vi "Standalone Status Monitor.vi"(11 "configuration file path":path) -> ()   [LabVIEW 2017, in "Status Monitor Library.lvlib"]
doc: "Use this template to build a producer/consumer design pattern. Use this template when you need to execute a process, such as data analysis, when a data source, such as a triggered acquisition, produces data at an uneven rate and you need to execute the process when the data becomes available."
uses:
  Status Monitor Library.lvlib
  Communications/Communications Library.lvlib
  Network Shared Variables/Shared Variables Library.lvlib
panel:
  in  "Process Stop Button":bool
  out "Demuxing":bool
  out "Total Samples":i32
  out "Post-Buffered Samples":i32
  out "Pre-Buffered Samples":i32
  out "Device State":T1(ring)
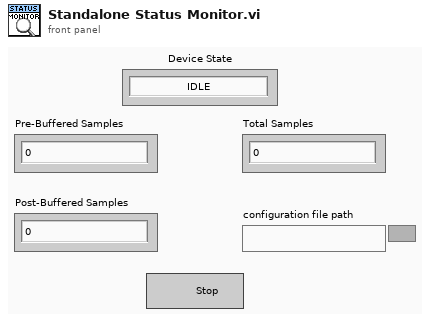
[diagram p1: front panel]
types:
  T1 = enum16{"IDLE", "ARM", "RUN_PRE-TRIGGER", "RUN_POST-TRIGGER", "POST_PROCESS", "CLEANUP"}
  T2 = typedef "Communications Library.lvlib/DTACQ Module Carrier Configuration--Cluster.ctl" = cluster{"Name":string, "IP":string, "Control Port":i32, "Timeout (ms)":i32, "Continuous Capture Port (Multiplexed)":i32, "Start HIL Shot Port":i32, "AWG Upload Port (Multiplexed)":i32, "Download Captured Data Port (Multiplexed)":i32, "Module Slots":i32, "Module Configurations":T3[]}
  T3 = typedef "Communications Library.lvlib/DTACQ Module Configuration--Cluster.ctl" = cluster{"Name":string, "Position":string, "Module Type":T4, "Control Port":i32, "Timeout (ms)":i32, "Channels":i32}
  T4 = typedef "Communications Library.lvlib/DTACQ Device Type--Enum.ctl" = enum16{"Carrier", "Analog In Module", "Analog Out Module", "Generic Module"}
  T5 = typedef "Communications Library.lvlib/DTACQ Connection Data--Cluster.ctl" = cluster{"Description":string, "Address":string, "Port":u16, "timeout (ms)":i32, "Termination Character":string, "TCP Connection Reference":refnum<k5>, "Open Connection":bool}
  T6 = typedef "Communications Library.lvlib/DTACQ Module Carrier Status.ctl" = cluster{"DTACQ State":T7, "Pre-Trigger Samples":i32, "Post-Trigger Samples":i32, "Total Samples":i32, "Post Processing":bool}
  T7 = typedef "Communications Library.lvlib/DTACQ Status--Enum.ctl" = enum16{"IDLE", "ARM", "RUN_PRE-TRIGGER", "RUN_POST-TRIGGER", "POST_PROCESS", "CLEANUP"}
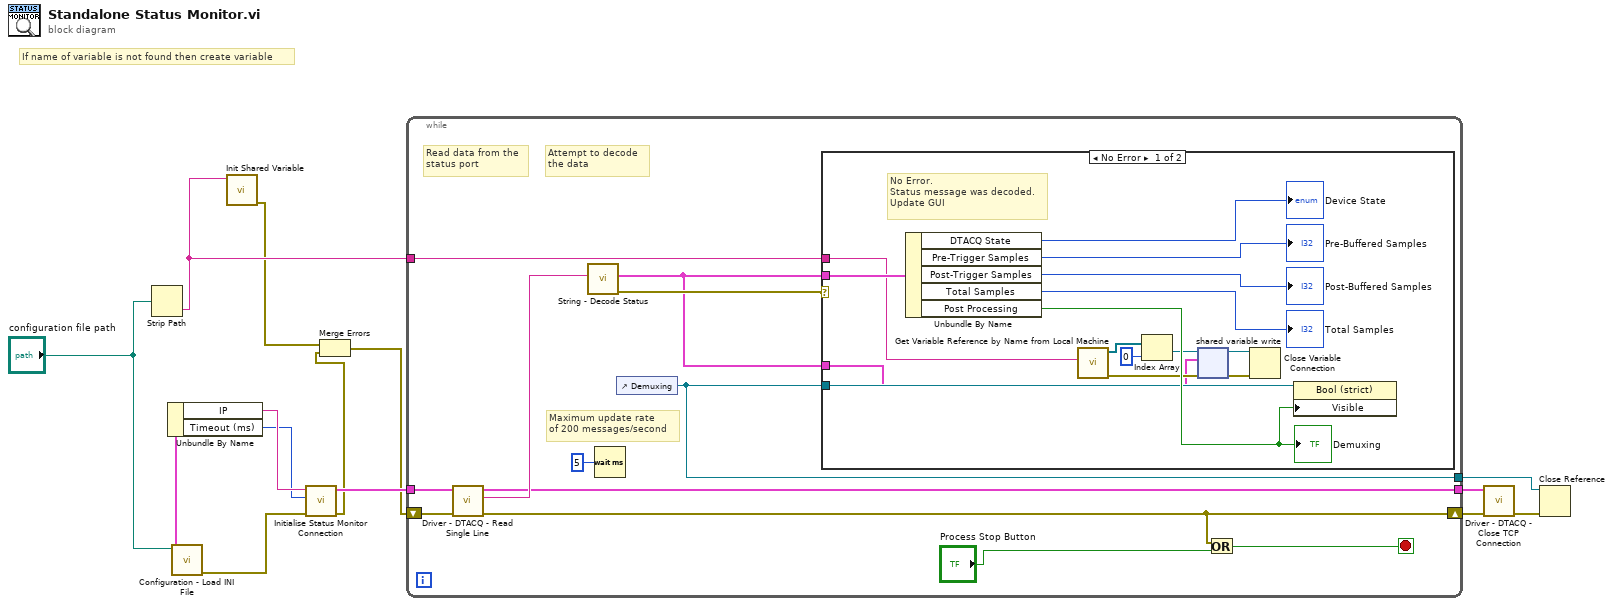
[diagram p0: block diagram]
diagram:
  # "If name of variable is not found then create variable"
  n1 = Strip Path(path="configuration file path") -> (name=w4:string)  [unwired: 1 out]
  n2 = call "Configuration - Load INI File.vi"("configuration file path"="configuration file path") -> ("error out"=w7:errorcluster, "Carrier Configuration Out"=w9:T2)  [unwired: 9 in]
  n3 = Unbundle By Name(w9) -> ("IP"=w8:string, "Timeout (ms)"=w6:i32)
  n4 = call "Init Shared Variable.vi"("name"=w4) -> ("error out 2"=w3:errorcluster)  [unwired: 10 in]
  n5 = call "Initialise Status Monitor Connection.vi"("error in"=w7, "timeout (ms)"=w6, "Address"=w8) -> ("error out"=w2:errorcluster, "Status Connection Out"=w14:T5)  [unwired: 7 in]
  n6 = Merge Errors(w3, w2) -> (w1:errorcluster)
  n7 = while {
    tunnel: w14 -> [w26]
    shift-right: [w22] -> w12
    shift-left: w1 -> [w24]
    tunnel: [w19] -> w13
    tunnel: [w18] -> w11
    tunnel: w4 -> [w15]
    stop <- w21 stop-if-true
    # "Maximum update rate\nof 200 messages/second"
    # "Attempt to decode\nthe data"
    # "Read data from the\nstatus port"
    n8 = call "Driver - DTACQ - Read Single Line.vi"("error in"=w24, "DTACQ Connection Data In"=w26) -> ("error out"=w22:errorcluster, "Read String"=w25:string, "DTACQ Connection Data Out"=w18:T5)  [unwired: 6 in, 1 out]
    n9 = call "String - Decode Status.vi"("Status Response String"=w25) -> ("error out"=w23:errorcluster, "Module Carrier Status"=w16:T6)  [unwired: 9 in]
    n10 = Wait (ms)(milliseconds to wait=u32 5) -> ()  [unwired: 1 out]
    n11 = control-ref of="Demuxing"() -> (w19:refnum<vi>)
    n12 = case shown="No Error" w23 {
      tunnel: w16 -> [w41 _]
      tunnel: w19 -> [w35 _]
      tunnel: w16 -> [w30 _]
      tunnel: w15 -> [w29 _]
      frame No Error {
        # "No Error.\nStatus message was decoded.\nUpdate GUI"
        n13 = Unbundle By Name(w41) -> ("DTACQ State"=→"Device State":T7, "Pre-Trigger Samples"=→"Pre-Buffered Samples":i32, "Post-Trigger Samples"=→"Post-Buffered Samples":i32, "Total Samples"=→"Total Samples":i32, "Post Processing"=w36:bool)
        "Demuxing" <- w36
        n14 = call "Get Variable Reference by Name from Local Machine.vi"("Search"=w29) -> ("error out"=w31:errorcluster, "Variable References Out"=w34:refnum<k21>[])  [unwired: 8 in, 1 out]
        n15 = Index Array(array=w34, index=0) -> (element=w33:refnum<k21>)
        n16 = shared-variable-write(w33, w31, w30) -> (w27:refnum<k21>, w28:errorcluster)
        n17 = Close Variable Connection(8:w28, 11:w27) -> ()  [unwired: 1 out]
        n18 = property class="Bool (strict)"(reference=w35, "Visible"=w36) -> ()  [unwired: 1 in, 2 out]
      }
      frame Error {
        # "Error decoding message.\nNot a valid status message,\nso leave the GUI as-is"
      }
    }
    n19 = Or(x=w22, y="Process Stop Button") -> (x .or. y?=w21:bool)
  }
  n20 = call "Driver - DTACQ - Close TCP Connection.vi"("error in"=w12, "DTACQ Connection Data In"=w11) -> ("error out"=w10:errorcluster)  [unwired: 8 in, 1 out]
  n21 = Close Reference(reference=w13, error in (no error)=w10) -> ()  [unwired: 1 out]
